vi "niFpgaDiscreteNormalizedIntegratorTemplate.vi"(0 "input":fxp<+/-,8,8>, 1 "reset":bool, 7 "initial condition":fxp<+/-,32,32>) -> (4 "output":fxp<+/-,32,32>)   [LabVIEW 2017]
doc: "Integrates a discrete input signal using forward Euler integration. The VI assumes that the integration interval (dt) is normalized to 1. The data type you wire to <B>input</B> determines <B>output</B> data type, where output word length is equal to input word length + 16 bits."
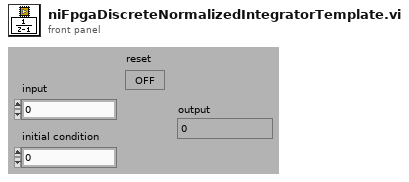
[diagram p1: front panel]
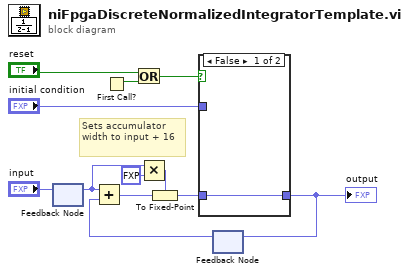
[diagram p0: block diagram]
diagram:
  # "Sets accumulator\nwidth to input + 16"
  n1 = feedback-in #1("input") -> ()
  n2 = feedback #1() -> (w3:fxp<+/-,8,8>)  [unwired: 1 in]
  n3 = First Call?() -> (First Call?: T/F=w7:bool)
  n4 = Or(x="reset", y=w7) -> (x .or. y?=w6:bool)
  n5 = Multiply(x=w3, y=fxp<+/-,16,16> 0.0) -> (x*y=w2:fxp<+/-,24,24>)
  n6 = feedback #2() -> (w11:fxp<+/-,32,32>)  [unwired: 1 in]
  n7 = Add(x=w3, y=w11) -> (x+y=w12:fxp<+/-,33,33>)
  n8 = To Fixed-Point(fixed-point type=w2, number=w12) -> (fixed-point=w9:fxp<+/-,24,24>)
  n9 = case shown="False" w6 {
    tunnel: "initial condition" -> [_ w14]
    tunnel: [w13 w14] -> w5
    tunnel: w9 -> [w13 _]
    frame False {
    }
    frame True {
      # "init or first call"
    }
  }
  "output" <- w5
  n10 = feedback-in #2(w5) -> ()
